vi "ElevatorControl.vi"() -> ()   [LabVIEW 2017, in "Thermal Shock.lvlib"]
uses:
  Thermal Shock.lvlib
  <vilib>/Instr/_visa.llb/VISA Configure Serial Port (Instr).vi
panel:
  out "error out":errorcluster
  in  "error in (no error)":errorcluster
  out "VISA resource name out":refnum<visa-resource-name>
  in  "VISA resource name":refnum<visa-resource-name>="LPT1"
  in  "Current State":bool
  out "Elevator Down":bool
  out "Elevator Up":bool
  in  "Stop":bool
  in  "Toggle Elevator!":bool
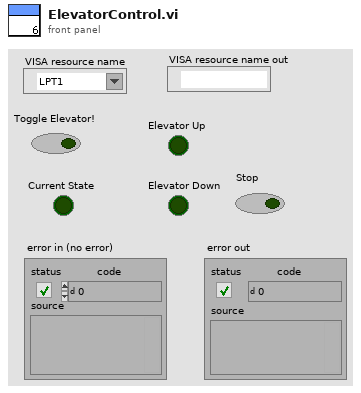
[diagram p1: front panel]
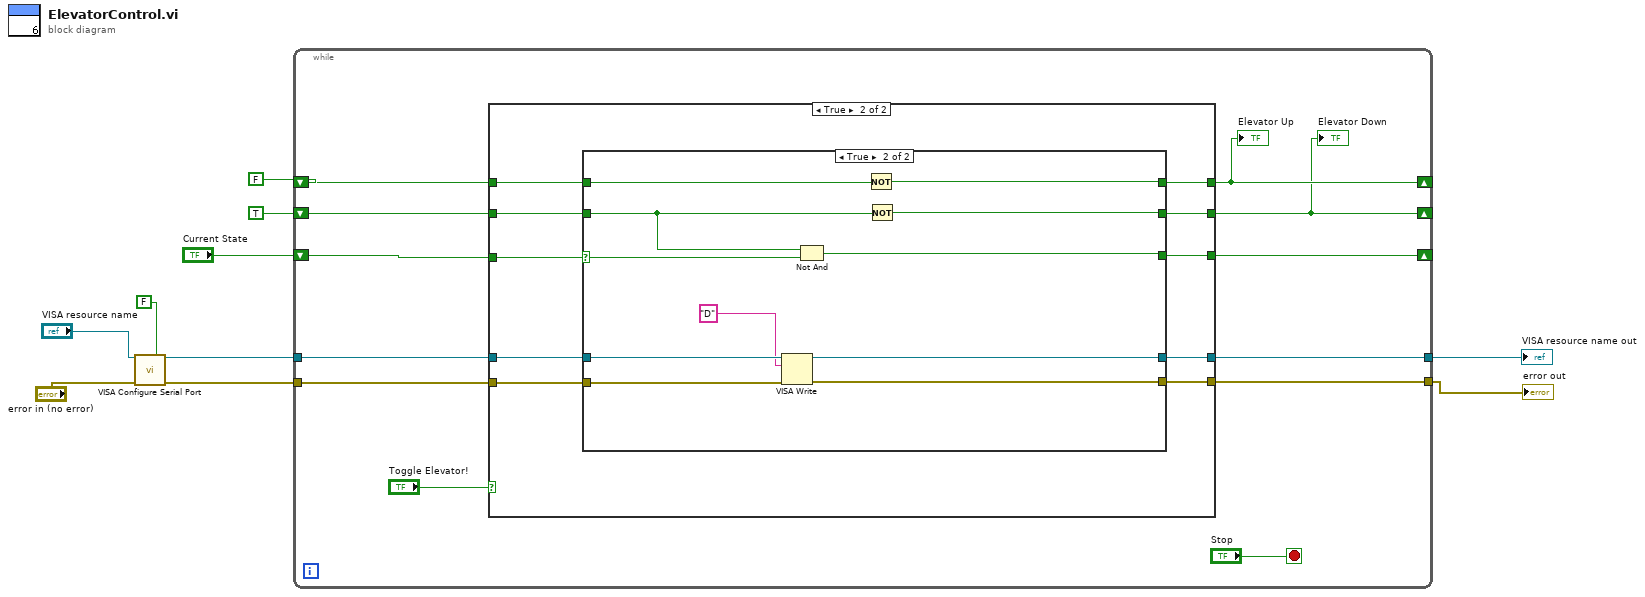
[diagram p0: block diagram]
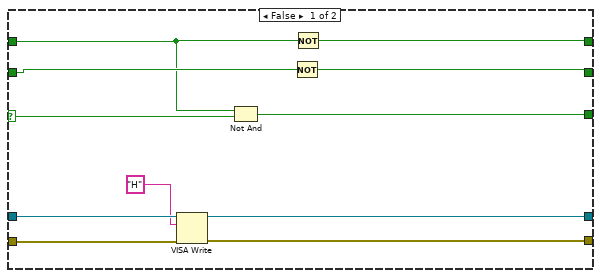
[diagram p3: hidden frame]
diagram:
  n1 = call-poly "VISA Configure Serial Port"("VISA resource name"="VISA resource name", "Enable Termination\nChar (T)"=FALSE, "error in (no error)"="error in (no error)") -> ("VISA resource name out"=w5:refnum<visa-resource-name>, "error out"=w3:errorcluster)  [unwired: 11 in]
  n2 = while {
    shift-right: [w16] -> _
    shift-left: FALSE -> [w20]
    shift-right: [w15] -> _
    shift-left: TRUE -> [w19]
    shift-right: [w17] -> _
    shift-left: "Current State" -> [w18]
    tunnel: w5 -> [w14]
    tunnel: w3 -> [w13]
    tunnel: [w12] -> w2
    tunnel: [w11] -> w1
    stop <- "Stop" stop-if-true
    n3 = case shown="True" "Toggle Elevator!" {
      tunnel: w20 -> [w26 w35]
      tunnel: w19 -> [w25 w34]
      tunnel: w18 -> [w27 w37]
      tunnel: [w27 w36] -> w17
      tunnel: [w26 w33] -> w16
      tunnel: [w25 w32] -> w15
      tunnel: w14 -> [w24 w31]
      tunnel: w13 -> [w23 w30]
      tunnel: [w24 w29] -> w12
      tunnel: [w23 w28] -> w11
      frame False {
      }
      frame True {
        n4 = case shown="True" w37 {
          selector: w37 -> [w48 w59]
          tunnel: [w47 w58] -> w36
          tunnel: w35 -> [w44 w57]
          tunnel: w34 -> [w46 w55]
          tunnel: [w43 w56] -> w33
          tunnel: [w45 w54] -> w32
          tunnel: w31 -> [w42 w53]
          tunnel: w30 -> [w41 w52]
          tunnel: [w39 w51] -> w29
          tunnel: [w40 w50] -> w28
          frame False {
            n5 = VISA Write(VISA resource name=w42, write buffer="H", error in (no error)=w41) -> (VISA resource name out=w39:refnum<visa-resource-name>, error out=w40:errorcluster)  [unwired: 1 out]
            n6 = Not And(1:w48, 2:w44) -> (0:w47:bool)
            n7 = Not(x=w46) -> (.not. x?=w45:bool)
            n8 = Not(x=w44) -> (.not. x?=w43:bool)
          }
          frame True {
            n9 = VISA Write(VISA resource name=w53, write buffer="D", error in (no error)=w52) -> (VISA resource name out=w51:refnum<visa-resource-name>, error out=w50:errorcluster)  [unwired: 1 out]
            n10 = Not And(1:w59, 2:w55) -> (0:w58:bool)
            n11 = Not(x=w57) -> (.not. x?=w56:bool)
            n12 = Not(x=w55) -> (.not. x?=w54:bool)
          }
        }
      }
    }
    "Elevator Up" <- w16
    "Elevator Down" <- w15
  }
  "VISA resource name out" <- w2
  "error out" <- w1
